vi "CSM Reuse Module.vi"(5 "Init State (\"Macro: Initialize\")":string="Macro: Initialize", 7 "Name (\"\" to Use UUID)":string="Reuse Module") -> ()   [LabVIEW 2017, in "1. Create a reuse Module.lvlib"]
doc: "------------- lvcsm -------------\n[CSMStates]\nItem 0 = \"Event Structure\"\nItem 1 = \"Idle\"\nItem 2 = \"CSM Documentation\"\nItem 3 = \"VI Reference\"\nItem 4 = \"Error Handler\"\nItem 5 = \"Critical Error\"\nItem 6 = \"Target Error\"\nItem 7 = \"Target Timeout Error\"\nItem 8 = \"Async Response\"\nItem 9 = \"Response\"\nItem 10 = \"Async Message Posted\"\nItem 11 = \"Initialize Core Data\"\nItem 12 = \"Exit\"\nItem 13 = \"Data: Initialize\"\nItem 14 = \"Data: Cleanup\"\nItem 15 = \"Events: Register\"\nItem 16 = \"Events: Unregister\"\nItem 17 = \"UI: Initialize\"\nItem 18 = \"UI: Cursor Set\"\nItem 19 = \"UI: Front Panel State\"\nItem 20 = \"Macro: Initialize\"\nItem 21 = \"Macro: Exit\"\nItem 22 = \"API: Start\"\nItem 23 = \"API: Stop\"\nItem 24 = \"API: Set Level\"\nItem 25 = \"API: Get Level\"\nItem 26 = \"DoSth: Check If Greater than 0.5\"\n\n[CSMStatus]\nItem 0 = \"Error Occurred@Error Handler\"\nItem 1 = \"Check Started@API: Start\"\nItem 2 = \"Check Stoppped@API: Stop\""
uses:
  1. Create a reuse Module.lvlib
  user.lib/_NEVSTOP/Communicable State Machine(CSM)/AdvanceAPI/CSM - Break Down Multiple States String.vi
  user.lib/_NEVSTOP/Communicable State Machine(CSM)/AdvanceAPI/CSM - Compact Multiple States.vi
  user.lib/_NEVSTOP/Communicable State Machine(CSM)/AdvanceAPI/CSM - Make String Arguments Safe.vi
  user.lib/_NEVSTOP/Communicable State Machine(CSM)/AdvanceAPI/CSM - Keywords.vi
  user.lib/_NEVSTOP/Communicable State Machine(CSM)/Communicable State Machine.lvlib
panel:
  in  "Level":dbl=0.5 min=0.0 max=1.0 step=0.1 format="%#_13g"
  in  "Stop":bool
  in  "Start":bool
  out "publish status":bool
  out "Random":dbl
  out "State History":string
  # "Creating a reusable module typically does not require message interaction with other modules; it only needs to provide an external interface and publish the state of the module. Therefore, as long as these two aspects are clearly described, one can call the reusable module without understanding its internal implementation details. \n\nIn CSM modules, all cases can be considered as messages for invocation, but it is recommended to use API category as external interfaces. When sending status updates, notify external entities of changes by sending either Status or Interrupt Status. \n\nThe core functionality of this module is to randomly generate data every second and compare it with a threshold value.\n\nAPI: \n1. API: Set Level, with the parameter as a DBL string. Functionality: Configure threshold value.\n2. API: Get Level, without any parameters. Functionality: Retrieve current threshold configuration.\n3. API: Start, without any parameters. Functionality: Initiate random number comparison feature.\n4. API: Stop, without any parameters. Functionality: Cease random number comparison feature.\n\nStatus:\n1. Status Changed, with the parameter as the value of the random number generated when it exceeds 0.5"
  # "If"
  # ">"
  # ", Then"
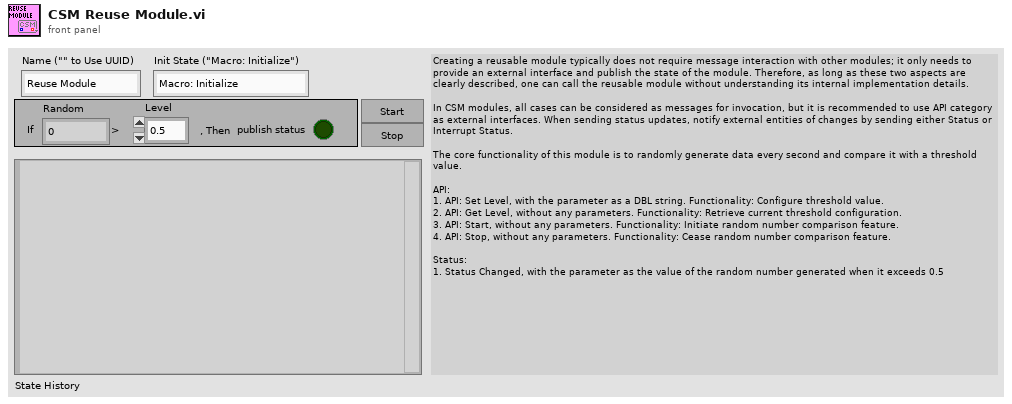
[diagram p1: front panel]
types:
  T1 = enum32{"Invalid", "Standard", "Closed", "Hidden", "Minimized", "Maximized"}
  T2 = enum32{"invalid app kind", "Development System", "Run Time System", "Student Edition", "Embedded LabVIEW", "Evaluation", "Custom"}
  T3 = typedef "Communicable State Machine.lvlib/_CSM_Response Source Message.ctl" = cluster{"‘State":string, "’Arguments":string, "’Error":errorcluster}
  T4 = cluster{"Current VI Reference":refnum<vi>, "Close Panel on Exit?":bool}
  T5 = cluster{"Core":cluster{"Current VI Reference":refnum<vi>, "Close Panel on Exit?":bool}, "Your Boolean data":bool, "Your string data":string, "Level":dbl}
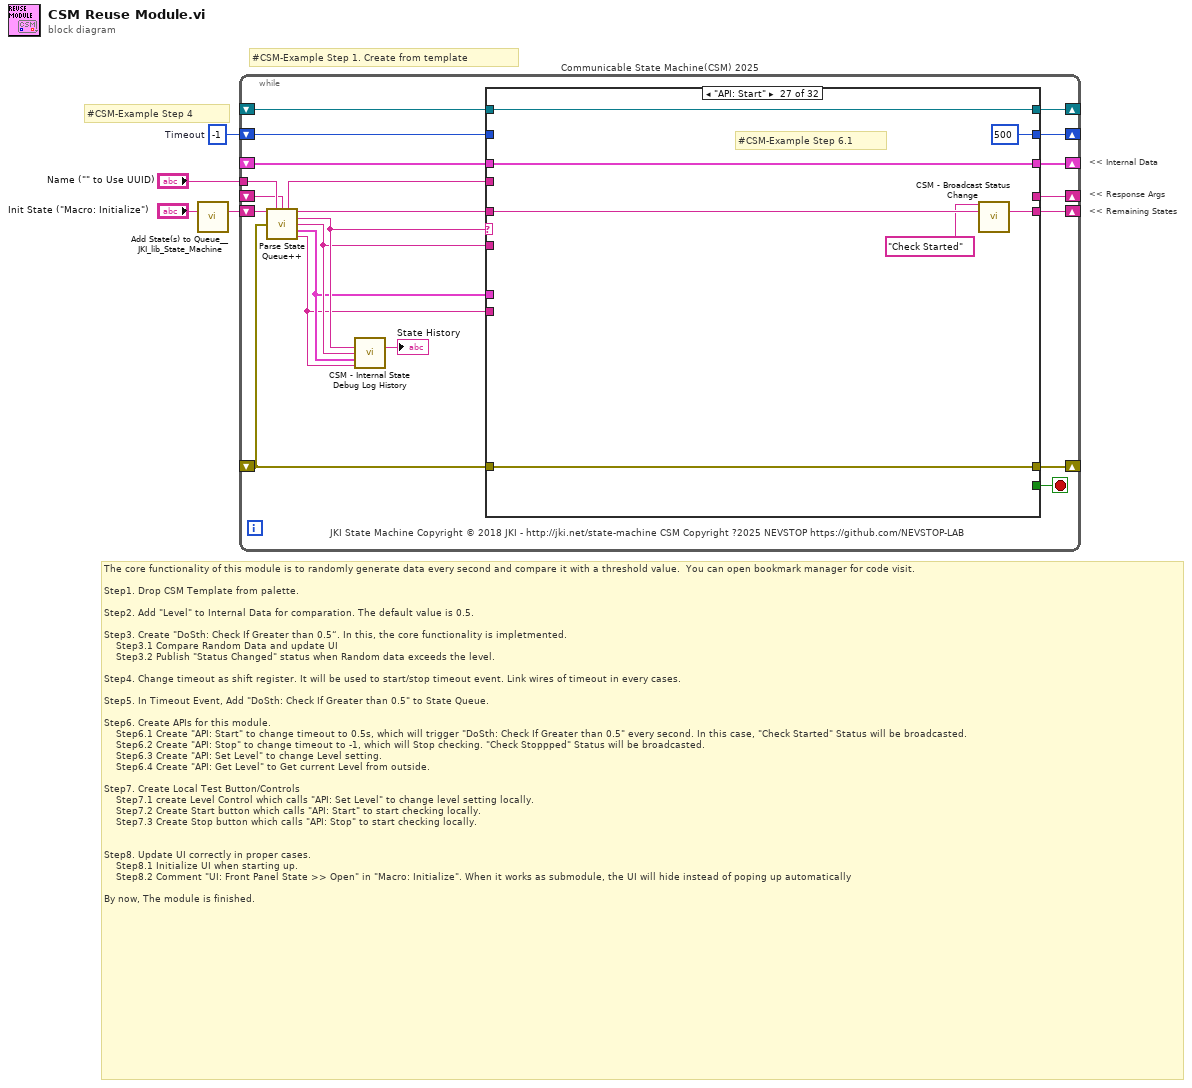
[diagram p0: block diagram]
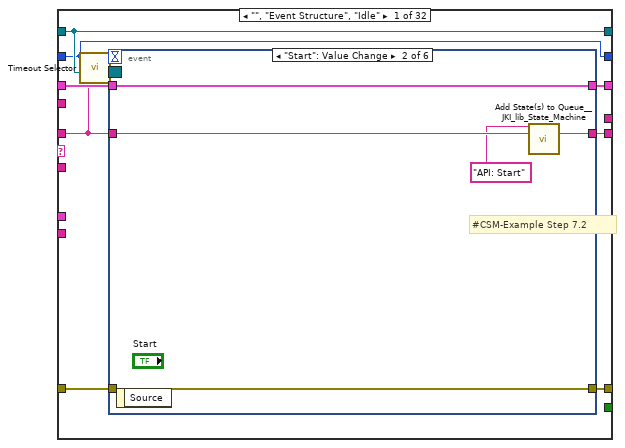
[diagram p2: hidden frame]
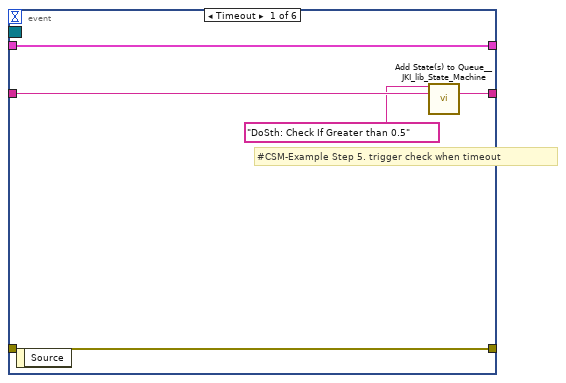
[diagram p3: hidden frame]
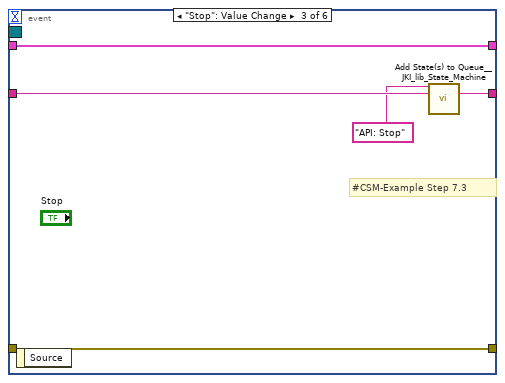
[diagram p4: hidden frame]
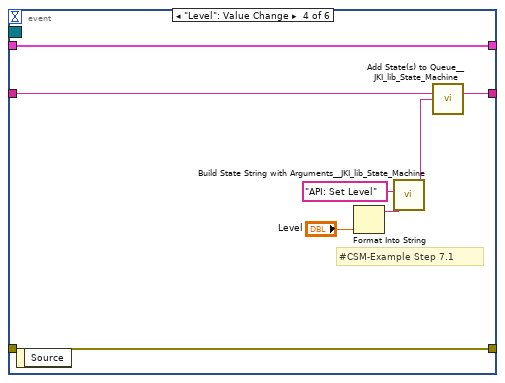
[diagram p5: hidden frame]
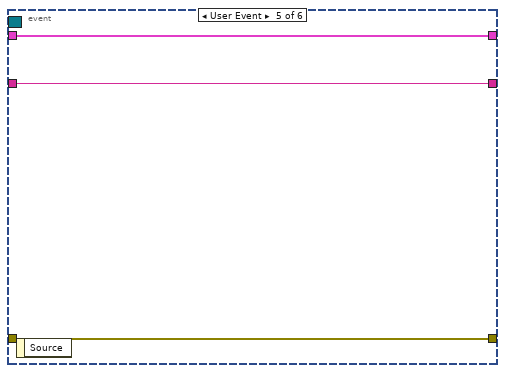
[diagram p6: hidden frame]
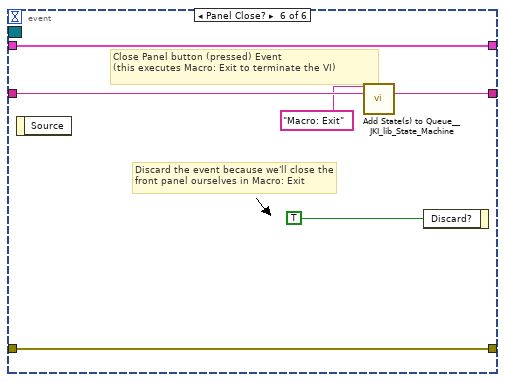
[diagram p7: hidden frame]
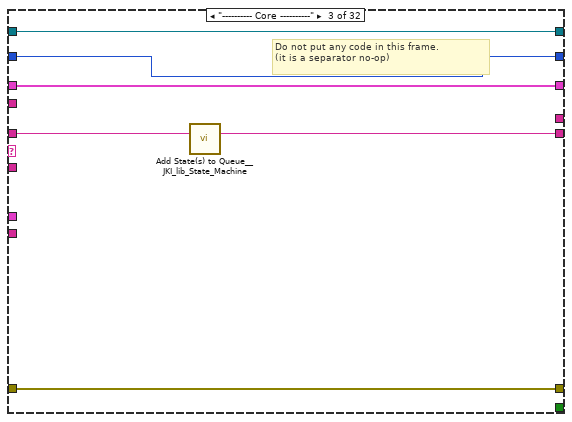
[diagram p9: hidden frame]
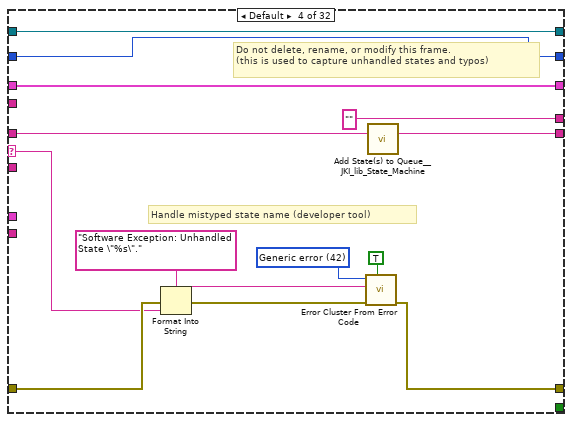
[diagram p10: hidden frame]
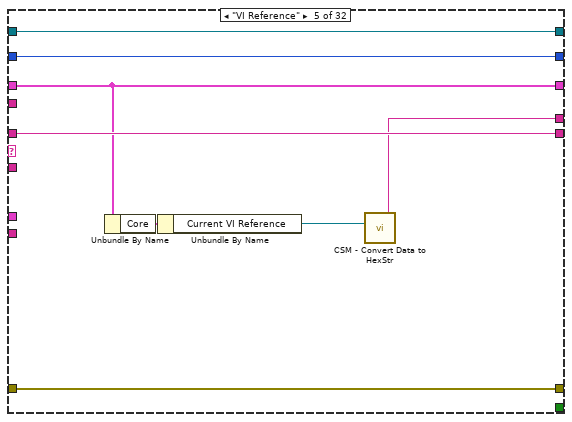
[diagram p11: hidden frame]
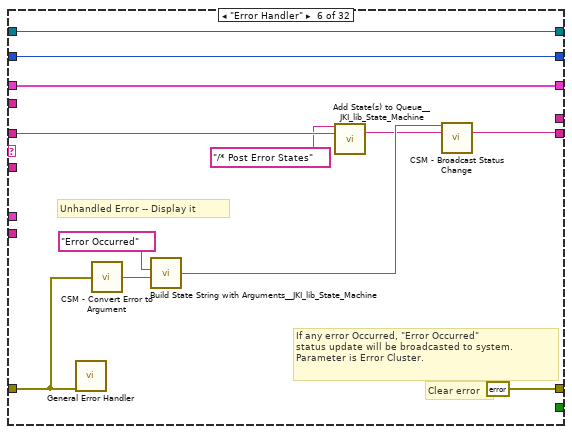
[diagram p12: hidden frame]
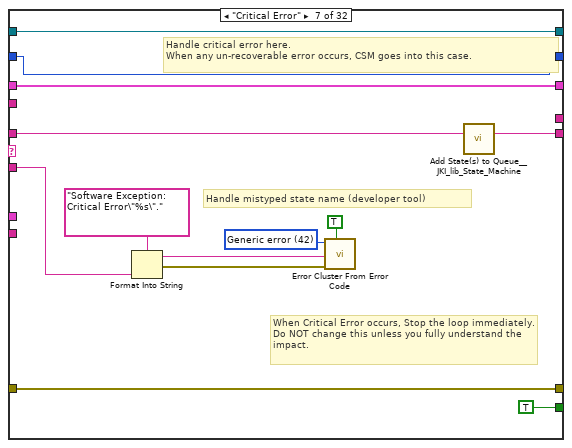
[diagram p13: hidden frame]
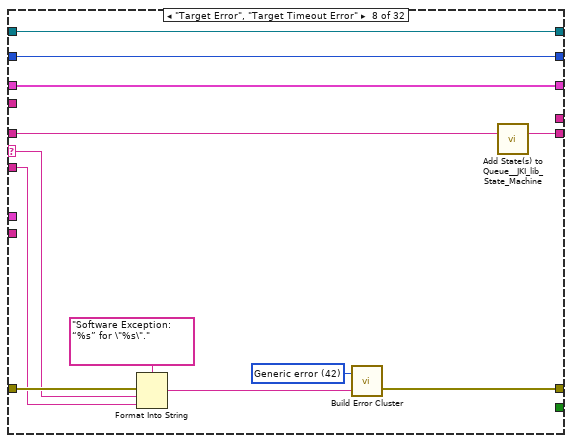
[diagram p14: hidden frame]
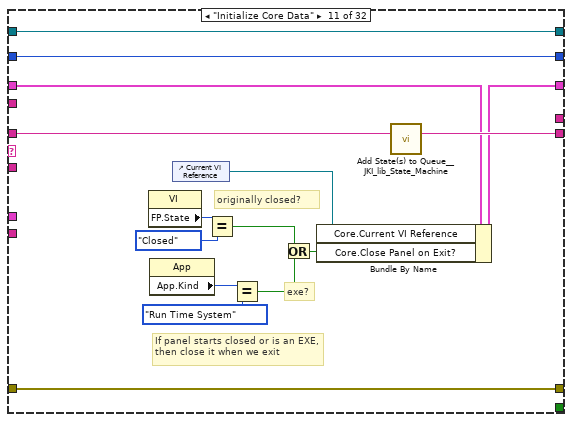
[diagram p17: hidden frame]
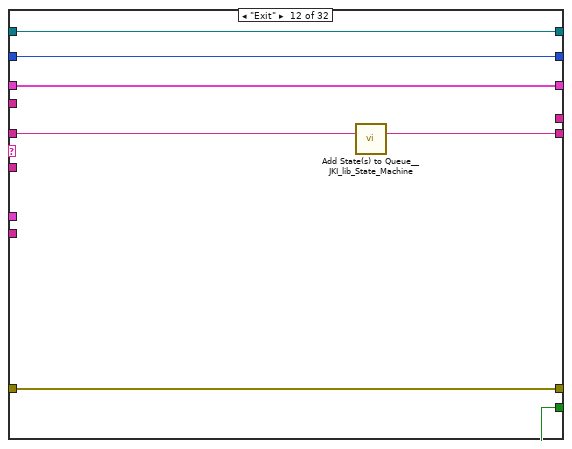
[diagram p18: hidden frame]
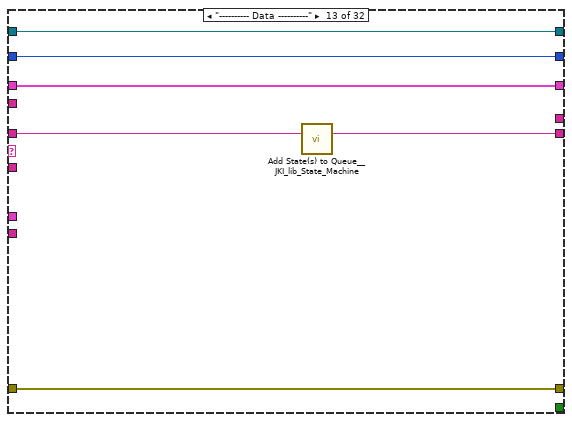
[diagram p19: hidden frame]
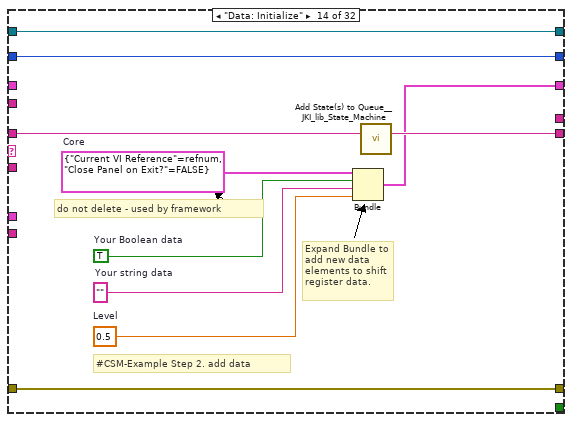
[diagram p20: hidden frame]
diagram:
  w2 = -1  # Timeout
  # "#CSM-Example Step 4"
  # "#CSM-Example Step 1. Create from template"
  # "The core functionality of this module is to randomly generate data every second and compare it with a threshold value.  You can open bookmark manager for code visit.\n\nStep1. Drop CSM Template from palette.\n\nStep2. Add \"Level\" to Internal Data for comparation. The default value is 0.5.\n\nStep3. Create \"DoSth: Check If Greater than 0.5“. In this, the core functionality is impletmented. \n    Step3.1 Compare Random Data and update UI\n    Step3.2 Publish \"Status Changed\" status when Random data exceeds the level.\n\nStep4. Change timeout as shift register. It will be used to start/stop timeout event. Link wires of timeout in every cases. \n\nStep5. In Timeout Event, Add \"DoSth: Check If Greater than 0.5\" to State Queue.\n\nStep6. Create APIs for this module.\n    Step6.1 Create \"API: Start\" to change timeout to 0.5s, which will trigger \"DoSth: Check If Greater than 0.5\" every second. In this case, \"Check Started\" Status will be broadcasted.\n    Step6.2 Create \"API: Stop\" to change timeout to -1, which will Stop checking. \"Check Stoppped\" Status will be broadcasted.\n    Step6.3 Create \"API: Set Level\" to change Level setting.\n    Step6.4 Create \"API: Get Level\" to Get current Level from outside.\n\nStep7. Create Local Test Button/Controls \n    Step7.1 create Level Control which calls \"API: Set Level\" to change level setting locally.\n    Step7.2 Create Start button which calls \"API: Start\" to start checking locally.\n    Step7.3 Create Stop button which calls \"API: Stop\" to start checking locally.\n    \n\nStep8. Update UI correctly in proper cases.\n    Step8.1 Initialize UI when starting up.\n    Step8.2 Comment \"UI: Front Panel State >> Open\" in \"Macro: Initialize\". When it works as submodule, the UI will hide instead of poping up automatically\n\nBy now, The module is finished."
  # "<< Internal Data"
  # "<< Response Args"
  # "<< Remaining States"
  n1 = call <vilib>:"Add State(s) to Queue__JKI_lib_State_Machine.vi"("State(s) in (\"\")"="Init State (\"Macro: Initialize\")") -> ("States Out"=w4:string)  [unwired: 14 in]
  n2 = while "Communicable State Machine(CSM) 2025" {
    shift-right: [w20] -> _
    shift-left: _ -> [w19]
    shift-right: [w23] -> _
    shift-left: _ -> [w18]
    shift-right: [w22] -> _
    shift-left: w4 -> [w24]
    tunnel: "Name (\"\" to Use UUID)" -> [w14]
    shift-right: [w17] -> _
    shift-left: _ -> [w8]
    shift-right: [w16] -> _
    shift-left: _ -> [w15]
    shift-right: [w6] -> _
    shift-left: w2 -> [w7]
    stop <- w21 stop-if-true
    # "JKI State Machine Copyright © 2018 JKI - http://jki.net/state-machine CSM Copyright ?2025 NEVSTOP https://github.com/NEVSTOP-LAB"
    n3 = call "Parse State Queue++.vi"("State Queue"=w24, "Name (\"\" to Use UUID)"=w14, "Response Arguments"=w8, "Previous Error"=w18) -> ("Name Used"=w9:string, "Remaining States"=w25:string, "Current State"=w13:string, "Arguments"=w12:string, ">> Response Source Message >>"=w11:T3, ">> Source CSM >>"=w10:string)  [unwired: 6 in]
    n4 = call "CSM - Internal State Debug Log History.vi"("State"=w13, "Arguments (\"\")"=w12, ">> Response Source Message >>"=w11, "Source (\"\")"=w10) -> ("Debug Log"=→"State History":string)  [unwired: 11 in]
    n5 = case shown="\"API: Start\"" w13 {
      selector: w13 -> [_ _ _ w81 _ _ _ w126 _ _ _ _ _ _ _ _ _ _ _ _ _ _ _ _ _ _ _ _ _ _ _ _]
      tunnel: w25 -> [w27 w70 w77 w85 w98 w111 w122 w128 w140 w145 w161 w168 w174 w184 w192 w198 w205 w210 w217 w224 w232 w249 w320 w327 w339 w343 w350 w357 w365 w372 w379 w393]
      tunnel: w12 -> [_ _ _ _ _ _ w115 w127 _ _ _ _ _ _ _ _ _ _ _ _ w227 w243 _ _ _ _ _ _ w360 _ _ _]
      tunnel: w19 -> [w33 w69 w74 w83 w97 w109 w123 w130 w139 w144 w154 w166 w171 _ w187 w195 w204 w209 w214 w219 w230 w245 w317 w324 w336 w342 w349 w356 w364 w369 w376 w384]
      tunnel: [w32 w71 w75 w87 w99 errorcluster {"status"=FALSE, "code"=0, "source"=""} ("error out") w124 w133 w141 w146 w158 w165 w172 w181 w188 w196 w200 w208 w215 w222 w228 w246 w318 w325 w337 w344 w351 w358 w366 w373 w377 w391] -> w23
      tunnel: w18 -> [w31 w71 w75 w86 w99 w100 w124 w132 w141 w146 w158 w165 w172 w181 w189 w196 _ w211 w215 w222 w229 w247 w318 w325 w337 w344 w351 w358 w366 w373 w377 w391]
      tunnel: [w34 w70 w76 w84 w98 w102 w121 w131 w140 w145 w160 w167 w173 w183 w191 w197 w205 w210 w216 w223 w231 w248 w319 w326 w338 w343 w346 w353 w365 w372 w378 w392] -> w22
      tunnel: [_ _ _ _ _ _ TRUE _ _ _ _ TRUE _ _ _ _ _ _ _ _ _ _ _ _ _ _ _ _ _ _ _ _] -> w21
      tunnel: [w30 w69 w74 w83 w97 w109 w123 w130 w139 w144 w159 w166 w171 w182 w187 w195 w204 w209 w214 w219 w230 w245 w317 w324 w336 w342 w349 w356 w361 w369 w376 w384] -> w20
      tunnel: w7 -> [w26 w67 w72 w78 w95 w101 w112 w125 w137 w142 w147 w162 w169 w176 w185 w193 w199 w206 w212 w220 w225 w241 w315 w321 w328 w340 _ _ w362 w370 w374 w385]
      tunnel: w10 -> [_ _ _ _ _ _ _ _ _ _ _ _ _ _ _ _ _ _ _ _ _ _ _ _ _ _ _ _ _ _ _ _]
      tunnel: w11 -> [_ _ _ _ _ _ _ _ _ _ _ _ _ _ _ _ _ _ _ _ _ _ _ _ _ _ _ _ _ _ _ _]
      tunnel: [_ _ _ "" w92 _ _ _ _ _ _ _ _ _ _ _ _ _ _ _ _ _ _ _ _ _ _ _ _ w367 _ _] -> w17
      tunnel: [w29 w68 w73 w79 w96 w107 w113 w129 w138 w143 w148 w163 w170 w177 w186 w194 w203 w207 w213 w221 w226 w242 w316 w322 w329 w341 w348 w355 w363 w371 w375 w390] -> w16
      tunnel: w15 -> [w29 w68 w73 w79 w96 w107 w113 w129 w138 w143 w148 w163 w170 w177 w186 w194 _ w207 w213 w221 w226 w242 w316 w322 w329 w341 w348 w355 w363 w371 w375 w390]
      tunnel: w9 -> [_ _ _ _ _ _ _ _ _ _ _ _ _ _ _ _ w202 _ _ _ _ _ _ _ _ _ _ _ _ _ _ _]
      tunnel: [w26 w67 w72 w78 w95 w101 w112 w125 w137 w142 w147 w162 w169 w176 w185 w193 w199 w206 w212 w220 w225 w241 w315 w321 w328 w340 500 ("Timeout") -1 ("Timeout") w362 w370 w374 w385] -> w6
      frame "", "Event Structure", "Idle" {
        n6 = call "Timeout Selector.vi"("Remaining States"=w27, "Timeout Expected"=w26) -> ("Timeout"=w28:i32)  [unwired: 5 in]
        n7 = event shown="[1] \"Start\": Value Change" {
          selector: w29 -> [_ _ _ _ _ _]
          dyn-events: _ -> [_ _ _ _ _ _]
          timeout: w28 -> [_ _ _ _ _ _]
          tunnel: w27 -> [w39 w44 w49 w55 w59 w66]
          tunnel: [w38 w43 w48 w54 w59 w65] -> w34
          tunnel: w33 -> [w36 w41 w46 w56 w60 w63]
          tunnel: [w37 w42 w47 w57 w58 w64] -> w32
          tunnel: w31 -> [w37 w42 w47 w57 w58 w64]
          tunnel: [w36 w41 w46 w56 w60 w63] -> w30
          event Timeout {
            # "#CSM-Example Step 5. trigger check when timeout"
            n8 = event-data() -> ()  [unwired: 1 in, 1 out]
            n9 = call <vilib>:"Add State(s) to Queue__JKI_lib_State_Machine.vi"("State(s) in Front (\"\")"="DoSth: Check If Greater than 0.5" ("State(s) in Front (\"\")"), "State(s) in (\"\")"=w39) -> ("States Out"=w38:string)  [unwired: 13 in]
          }
          event "Start": Value Change {
            # "#CSM-Example Step 7.2"
            n10 = event-data() -> ()  [unwired: 1 in, 1 out]
            n11 = call <vilib>:"Add State(s) to Queue__JKI_lib_State_Machine.vi"("State(s) in Front (\"\")"="API: Start" ("State(s) in Front (\"\")"), "State(s) in (\"\")"=w44) -> ("States Out"=w43:string)  [unwired: 13 in]
          }
          event "Stop": Value Change {
            # "#CSM-Example Step 7.3"
            n12 = event-data() -> ()  [unwired: 1 in, 1 out]
            n13 = call <vilib>:"Add State(s) to Queue__JKI_lib_State_Machine.vi"("State(s) in Front (\"\")"="API: Stop" ("State(s) in Front (\"\")"), "State(s) in (\"\")"=w49) -> ("States Out"=w48:string)  [unwired: 13 in]
          }
          event "Level": Value Change {
            # "#CSM-Example Step 7.1"
            n14 = event-data() -> ()  [unwired: 1 in, 1 out]
            n15 = Format Into String("Level") -> (resulting string=w50:string)  [unwired: 3 in, 1 out]
            n16 = call <vilib>:"Build State String with Arguments__JKI_lib_State_Machine.vi"("Arguments (\"\")"=w50, "State"="API: Set Level") -> ("State with Arguments"=w53:string)  [unwired: 4 in]
            n17 = call <vilib>:"Add State(s) to Queue__JKI_lib_State_Machine.vi"("State(s) in (\"\")"=w55, "State(s) at Back (\"\")"=w53) -> ("States Out"=w54:string)  [unwired: 13 in]
          }
          event User Event {
            n18 = event-data() -> ()  [unwired: 1 in, 1 out]
          }
          event Panel Close? {
            # "Discard the event because we'll close the front panel ourselves in Macro: Exit"
            # "Close Panel button (pressed) Event\n(this executes Macro: Exit to terminate the VI)"
            n19 = event-data() -> ()  [unwired: 1 in, 1 out]
            n20 = call <vilib>:"Add State(s) to Queue__JKI_lib_State_Machine.vi"("State(s) in Front (\"\")"="Macro: Exit", "State(s) in (\"\")"=w66) -> ("States Out"=w65:string)  [unwired: 13 in]
            n21 = event-data("Discard?"=TRUE) -> ()  [unwired: 1 in, 1 out]
          }
        }
      }
      frame "CSM Documentation" {
        # "#CSM README FIRST\n\nCSM is a LabVIEW application framework that builds upon JKI State Machine (JKISM). It follows the pattern of JKISM and extends the keywords to describe message communication between CSM modules, including concepts such as Sync-Message, Async-Message, Subscription/Unsubscription of status - essential elements for creating reusable code modules. For more information, please visit the CSM wiki: https://github.com/NEVSTOP-LAB/JKI-State-Machine-Plus-Plus/wiki\n\nFor instructions on JKI State Machine, visit: http://jki.net/state-machine/\nFor information about CSM, visit: https://github.com/NEVSTOP-LAB"
        # "CSM Documentation"
      }
      frame "---------- Core ----------" {
        # "Do not put any code in this frame.\n(it is a separator no-op)"
        n22 = call <vilib>:"Add State(s) to Queue__JKI_lib_State_Machine.vi"("State(s) in (\"\")"=w77) -> ("States Out"=w76:string)  [unwired: 14 in]
      }
      frame Default {
        w90 = 42 items=["No error", "Argument error", "Memory is full", "Out of zone", "End of file", "File already open", "Generic file I/O error", "File not found", "File permission error", "Disk is full", "Duplicate path", "Too many files open", "System feature not enabled", "Resource file not found", "Cannot add resource", "Resource not found", "Image not found", "Image memory error", "Pen does not exist", "Config type invalid", "Config token not found", "Config parse error", "Config memory error", "Bad external code format", "Bad external code offset", "External code not present", "Null window", "Destroy window error", "Null menu", "Print aborted", "Bad print record", "Print driver error", "Windows error during printing", "Memory error during printing", "Print dialog error", "Generic print error", "Invalid device refnum", "Device not found", "Device parameter error", "Device unit error", "Cannot open device", "Device call aborted", "Generic error", "Cancelled by user", "Object ID too low", "Object ID too high", "Object not in heap", "Unknown heap", "Unknown object (invalid DefProc)", "Unknown object (DefProc not in table)", "Message out of range", "Invalid (null) method", "Unknown message", "Manager call not supported", "Bad address", "Network operation in progress", "Network operation timed out", "Connection is busy", "Network attribute not supported", "Network error", "Address in use", "System out of memory", "Connection aborted", "Connection refused", "Not connected", "Already connected", "Connection closed", "Initialization error (interapplication manager)", "Bad occurrence", "Wait on unbound occurrence handler", "Occurrence queue overflow", "Datalog type conflict", "Unused", "Unrecognized type (interapplication manager)", "Memory corrupt", "Failed to make temporary DLL", "Old CIN version", "Drag socket not found", "Failed to load drop-object", "Failed to register OLE object", "Failed to release OLE object", "Format specifier type mismatch", "Unknown format specifier", "Too few format specifiers", "Too many format specifiers", "Scan failed", "Newer CIN version", "Error converting to variant", "Runtime menu error", "Password tampered", "Variant attribute not found", "Incompatible variant data type", "Event data is not available", "Event Store is not present", "Occurrence is not found", "Event Queue is not created", "Event info is not available", "Refnum passed is NULL", "Error retrieving Class GUID", "Error retrieving CoClass GUID", "Error retrieving TypeLib GUID.", "Bad built application magic bytes.", "Specific driver is different from the specific driver associated with the Logical Name.", "There is no session opened to the class driver.", "Max Error", "MAX - Error with config objects", "MAX - Error loading configuration", "MAX - Group not supported"]
        # "Do not delete, rename, or modify this frame.\n(this is used to capture unhandled states and typos)"
        # "Handle mistyped state name (developer tool)"
        n23 = Format Into String(format string="Software Exception: Unhandled State \"%s\"." ("message"), error in=w86, w81) -> (resulting string=w89:string, error out=w88:errorcluster)  [unwired: 1 in]
        n24 = call <vilib>:"Error Cluster From Error Code.vi"("show call chain? (False)"=TRUE, "error in (no error)"=w88, "error message (\"\")"=w89, "error code (0)"=w90) -> ("error out"=w87:errorcluster)  [unwired: 5 in]
        n25 = call <vilib>:"Add State(s) to Queue__JKI_lib_State_Machine.vi"("State(s) in (\"\")"=w85) -> ("States Out"=w84:string)  [unwired: 14 in]
      }
      frame "VI Reference" {
        n26 = Unbundle By Name(w97) -> ("Core"=w94:T4)
        n27 = Unbundle By Name(w94) -> ("Current VI Reference"=w93:refnum<vi>)
        n28 = call "CSM - Convert Data to HexStr.vi"("Variant"=w93) -> ("HEX String (0-9,A-F)"=w92:string)  [unwired: 8 in]
      }
      frame "Error Handler" {
        # "If any error Occurred, \"Error Occurred\" \nstatus update will be broadcasted to system.\nParameter is Error Cluster."
        # "Unhandled Error -- Display it"
        # "Clear error"
        n29 = call <vilib>:"General Error Handler.vi"("error in (no error)"=w100) -> ()  [unwired: 10 in, 5 out]
        n30 = call "CSM - Convert Error to Argument.vi"("Error"=w100) -> ("Argument"=w105:string)  [unwired: 4 in]
        n31 = call <vilib>:"Build State String with Arguments__JKI_lib_State_Machine.vi"("Arguments (\"\")"=w105, "State"="Error Occurred" ("Status with Arguments")) -> ("State with Arguments"=w104:string)  [unwired: 4 in]
        n32 = call <vilib>:"Add State(s) to Queue__JKI_lib_State_Machine.vi"("State(s) in Front (\"\")"="/* Post Error States", "State(s) in (\"\")"=w111) -> ("States Out"=w103:string)  [unwired: 13 in]
        n33 = call "CSM - Broadcast Status Change.vi"("Status With Arguments"=w104, "State Queue"=w103) -> ("Remaining States"=w102:string)  [unwired: 13 in]
      }
      frame "Critical Error" {
        w119 = 42 items=["No error", "Argument error", "Memory is full", "Out of zone", "End of file", "File already open", "Generic file I/O error", "File not found", "File permission error", "Disk is full", "Duplicate path", "Too many files open", "System feature not enabled", "Resource file not found", "Cannot add resource", "Resource not found", "Image not found", "Image memory error", "Pen does not exist", "Config type invalid", "Config token not found", "Config parse error", "Config memory error", "Bad external code format", "Bad external code offset", "External code not present", "Null window", "Destroy window error", "Null menu", "Print aborted", "Bad print record", "Print driver error", "Windows error during printing", "Memory error during printing", "Print dialog error", "Generic print error", "Invalid device refnum", "Device not found", "Device parameter error", "Device unit error", "Cannot open device", "Device call aborted", "Generic error", "Cancelled by user", "Object ID too low", "Object ID too high", "Object not in heap", "Unknown heap", "Unknown object (invalid DefProc)", "Unknown object (DefProc not in table)", "Message out of range", "Invalid (null) method", "Unknown message", "Manager call not supported", "Bad address", "Network operation in progress", "Network operation timed out", "Connection is busy", "Network attribute not supported", "Network error", "Address in use", "System out of memory", "Connection aborted", "Connection refused", "Not connected", "Already connected", "Connection closed", "Initialization error (interapplication manager)", "Bad occurrence", "Wait on unbound occurrence handler", "Occurrence queue overflow", "Datalog type conflict", "Unused", "Unrecognized type (interapplication manager)", "Memory corrupt", "Failed to make temporary DLL", "Old CIN version", "Drag socket not found", "Failed to load drop-object", "Failed to register OLE object", "Failed to release OLE object", "Format specifier type mismatch", "Unknown format specifier", "Too few format specifiers", "Too many format specifiers", "Scan failed", "Newer CIN version", "Error converting to variant", "Runtime menu error", "Password tampered", "Variant attribute not found", "Incompatible variant data type", "Event data is not available", "Event Store is not present", "Occurrence is not found", "Event Queue is not created", "Event info is not available", "Refnum passed is NULL", "Error retrieving Class GUID", "Error retrieving CoClass GUID", "Error retrieving TypeLib GUID.", "Bad built application magic bytes.", "Specific driver is different from the specific driver associated with the Logical Name.", "There is no session opened to the class driver.", "Max Error", "MAX - Error with config objects", "MAX - Error loading configuration", "MAX - Group not supported"]
        # "Handle critical error here.\nWhen any un-recoverable error occurs, CSM goes into this case."
        # "When Critical Error occurs, Stop the loop immediately. Do NOT change this unless you fully understand the impact."
        # "Handle mistyped state name (developer tool)"
        n34 = Format Into String(format string="Software Exception: Critical Error\"%s\"." ("message"), w115) -> (resulting string=w118:string, error out=w117:errorcluster)  [unwired: 2 in]
        n35 = call <vilib>:"Error Cluster From Error Code.vi"("show call chain? (False)"=TRUE, "error in (no error)"=w117, "error message (\"\")"=w118, "error code (0)"=w119) -> ()  [unwired: 5 in, 1 out]
        n36 = call <vilib>:"Add State(s) to Queue__JKI_lib_State_Machine.vi"("State(s) in (\"\")"=w122) -> ("States Out"=w121:string)  [unwired: 14 in]
      }
      frame "Target Error", "Target Timeout Error" {
        w135 = 42 items=["No error", "Argument error", "Memory is full", "Out of zone", "End of file", "File already open", "Generic file I/O error", "File not found", "File permission error", "Disk is full", "Duplicate path", "Too many files open", "System feature not enabled", "Resource file not found", "Cannot add resource", "Resource not found", "Image not found", "Image memory error", "Pen does not exist", "Config type invalid", "Config token not found", "Config parse error", "Config memory error", "Bad external code format", "Bad external code offset", "External code not present", "Null window", "Destroy window error", "Null menu", "Print aborted", "Bad print record", "Print driver error", "Windows error during printing", "Memory error during printing", "Print dialog error", "Generic print error", "Invalid device refnum", "Device not found", "Device parameter error", "Device unit error", "Cannot open device", "Device call aborted", "Generic error", "Cancelled by user", "Object ID too low", "Object ID too high", "Object not in heap", "Unknown heap", "Unknown object (invalid DefProc)", "Unknown object (DefProc not in table)", "Message out of range", "Invalid (null) method", "Unknown message", "Manager call not supported", "Bad address", "Network operation in progress", "Network operation timed out", "Connection is busy", "Network attribute not supported", "Network error", "Address in use", "System out of memory", "Connection aborted", "Connection refused", "Not connected", "Already connected", "Connection closed", "Initialization error (interapplication manager)", "Bad occurrence", "Wait on unbound occurrence handler", "Occurrence queue overflow", "Datalog type conflict", "Unused", "Unrecognized type (interapplication manager)", "Memory corrupt", "Failed to make temporary DLL", "Old CIN version", "Drag socket not found", "Failed to load drop-object", "Failed to register OLE object", "Failed to release OLE object", "Format specifier type mismatch", "Unknown format specifier", "Too few format specifiers", "Too many format specifiers", "Scan failed", "Newer CIN version", "Error converting to variant", "Runtime menu error", "Password tampered", "Variant attribute not found", "Incompatible variant data type", "Event data is not available", "Event Store is not present", "Occurrence is not found", "Event Queue is not created", "Event info is not available", "Refnum passed is NULL", "Error retrieving Class GUID", "Error retrieving CoClass GUID", "Error retrieving TypeLib GUID.", "Bad built application magic bytes.", "Specific driver is different from the specific driver associated with the Logical Name.", "There is no session opened to the class driver.", "Max Error", "MAX - Error with config objects", "MAX - Error loading configuration", "MAX - Group not supported"]
        n37 = Format Into String(format string="Software Exception: “%s” for \"%s\"." ("message"), error in=w132, w126, w127) -> (resulting string=w134:string)  [unwired: 1 in, 1 out]
        n38 = call "Build Error Cluster.vi"("String to Prepend to Source (\"\")"=w134, "Code"=w135) -> ("error out"=w133:errorcluster)
        n39 = call <vilib>:"Add State(s) to Queue__JKI_lib_State_Machine.vi"("State(s) in (\"\")"=w128) -> ("States Out"=w131:string)  [unwired: 14 in]
      }
      frame "Async Response", "Response" {
        # "Handle Async-call Response (\"Async Response\" for ->)"
        # "Handle Sync-call Response (\"Response\" for @)"
        # "After Message is executed, CSM goes to this state for receive the response. \n    For Async Message(->), \"Async Response\" is used. This CSM will goes to \"Async Message Posted\" immediately and receive the \"Async Response\" after the callee finishes the message.\n    For Sync Message(@),  This CSM will wait until the message is done and immediately goes to \"Response\""
      }
      frame "Async Message Posted" {
        # "Handle post action for async message (->)."
        # "After Async Message is posted (->), CSM goes to this state for post-action. You can use Argument - State to tell which Async Message is called."
      }
      frame "Initialize Core Data" {
        # "originally closed?"
        # "exe?"
        # "If panel starts closed or is an EXE, then close it when we exit"
        n40 = property class="VI"() -> ("FP.State"=w151:T1)  [unwired: 2 in, 2 out]
        n41 = property class="App"() -> ("App.Kind"=w157:T2)  [unwired: 2 in, 2 out]
        n42 = control-ref of="Current VI Reference"() -> (w152:refnum<vi>)
        n43 = Equal?(x=w151, y=T1."Closed" ("Front Panel Window:State")) -> (x = y?=w149:bool)
        n44 = Equal?(x=w157, y=T2."Run Time System" ("Application:Kind")) -> (x = y?=w155:bool)
        n45 = Or(x=w149, y=w155) -> (x .or. y?=w153:bool)
        n46 = Bundle By Name(cluster=w154, "Core.Current VI Reference"=w152, "Core.Close Panel on Exit?"=w153) -> (w159:T5)
        n47 = call <vilib>:"Add State(s) to Queue__JKI_lib_State_Machine.vi"("State(s) in (\"\")"=w161) -> ("States Out"=w160:string)  [unwired: 14 in]
      }
      frame "Exit" {
        n48 = call <vilib>:"Add State(s) to Queue__JKI_lib_State_Machine.vi"("State(s) in (\"\")"=w168) -> ("States Out"=w167:string)  [unwired: 14 in]
      }
      frame "---------- Data ----------" {
        n49 = call <vilib>:"Add State(s) to Queue__JKI_lib_State_Machine.vi"("State(s) in (\"\")"=w174) -> ("States Out"=w173:string)  [unwired: 14 in]
      }
      frame "Data: Initialize" {
        w175 = 0.5  # Level
        w178 = T4 {"Current VI Reference"=refnum, "Close Panel on Exit?"=FALSE}  # Core
        w180 = TRUE  # Your Boolean data
        w179 = ""  # Your string data
        # "#CSM-Example Step 2. add data"
        # "do not delete - used by framework"
        # "Expand Bundle to add new data elements to shift register data."
        n50 = Bundle("Core"=w178, "Your Boolean data"=w180, "Your string data"=w179, "Level"=w175) -> (w182:T5)  [unwired: 1 in]
        n51 = call <vilib>:"Add State(s) to Queue__JKI_lib_State_Machine.vi"("State(s) in (\"\")"=w184) -> ("States Out"=w183:string)  [unwired: 14 in]
      }
      frame "Data: Cleanup" {
        n52 = Unbundle By Name(w187) -> ("Core.Current VI Reference"=w190:refnum<vi>)
        n53 = Close Reference(reference=w190, error in (no error)=w189) -> (error out=w188:errorcluster)
        n54 = call <vilib>:"Add State(s) to Queue__JKI_lib_State_Machine.vi"("State(s) in (\"\")"=w192) -> ("States Out"=w191:string)  [unwired: 14 in]
      }
      frame "---------- Events ----------" {
        n55 = call <vilib>:"Add State(s) to Queue__JKI_lib_State_Machine.vi"("State(s) in (\"\")"=w198) -> ("States Out"=w197:string)  [unwired: 14 in]
      }
      frame "Events: Register" {
        # "Register message event to break Waiting in Event structure."
        n56 = call "CSM - Get New State Notifier Event.vi"("Name (\"\" to Use UUID) In"=w202) -> ("error out"=w200:errorcluster, "New State Notifier Event"=w201:refnum<user-event>)  [unwired: 9 in]
        n57 = register-events(w201) -> (reference out=w203:refnum<event-registration>)  [unwired: 2 in, 1 out]
      }
      frame "Events: Unregister" {
        n58 = Unregister For Events(event registration refnum=w207, error in=w211) -> (error out=w208:errorcluster)
      }
      frame "---------- UI ----------" {
        n59 = call <vilib>:"Add State(s) to Queue__JKI_lib_State_Machine.vi"("State(s) in (\"\")"=w217) -> ("States Out"=w216:string)  [unwired: 14 in]
      }
      frame "UI: Initialize" {
        # "#CSM-Example Step 8.1"
        n60 = Unbundle By Name(w219) -> ("Level"=w218:dbl)
        n61 = local write "Level"(w218) -> ()
        n62 = call <vilib>:"Add State(s) to Queue__JKI_lib_State_Machine.vi"("State(s) in (\"\")"=w224) -> ("States Out"=w223:string)  [unwired: 14 in]
      }
      frame "UI: Cursor Set" {
        # "Argument"
        n63 = disable-structure shown="TARGET_TYPE!=Windows" {
          disable-tunnel: w229 -> [w235 w240]
          disable-tunnel: [w234 w240] -> w228
          disable-tunnel: w227 -> [w233 _]
          frame condition #0 (active) {
            n64 = case shown="\"Idle\", Default" w233 {
              tunnel: w235 -> [w237 w239]
              tunnel: [w236 w238] -> w234
              frame "Idle", Default {
                n65 = call <vilib>:"Unset Busy.vi"("error in (no error)"=w237) -> ("error out"=w236:errorcluster)  [unwired: 10 in]
              }
              frame "Busy" {
                n66 = call <vilib>:"Set Busy.vi"("error in (no error)"=w239) -> ("error out"=w238:errorcluster)  [unwired: 9 in, 1 out]
              }
            }
          }
          frame condition #1 {
          }
        }
        n67 = call <vilib>:"Add State(s) to Queue__JKI_lib_State_Machine.vi"("State(s) in (\"\")"=w232) -> ("States Out"=w231:string)  [unwired: 14 in]
      }
      frame "UI: Front Panel State" {
        # "Argument"
        n68 = Unbundle By Name(w245) -> ("Core.Current VI Reference"=w244:refnum<vi>)
        n69 = call <vilib>:"Add State(s) to Queue__JKI_lib_State_Machine.vi"("State(s) in (\"\")"=w249) -> ("States Out"=w248:string)  [unwired: 14 in]
        n70 = case shown="\"Close\", \"Closed\"" w243 {
          tunnel: w247 -> [w255 w270 w281 w294 w307]
          tunnel: [w257 w271 w283 w296 w309] -> w246
          tunnel: w244 -> [w256 w268 w282 w295 w308]
          frame "Open", "Standard", Default {
            w250 = T1."Standard" ("State")
            n71 = property class="VI"(reference=w256, error in=w255) -> (reference out=w253:refnum<vi>, error out=w254:errorcluster, "FP.State"=w252:T1)
            n72 = Not Equal?(x=w252, y=w250) -> (x != y?=w251:bool)
            n73 = case shown="True" w251 {
              tunnel: [w261 w263] -> w257
              tunnel: w254 -> [w260 w263]
              tunnel: w253 -> [w259 _]
              tunnel: w250 -> [w258 _]
              frame True {
                n74 = invoke class="VI" method="FP.Open"(reference=w259, error in=w260, "Activate"=TRUE, "State"=w258) -> (error out=w261:errorcluster)  [unwired: 1 in, 4 out]
              }
              frame False {
              }
            }
          }
          frame "Close", "Closed" {
            n75 = property class="VI"(reference=w268, error in=w270) -> (reference out=w267:refnum<vi>, error out=w269:errorcluster, "FP.State"=w265:T1)
            n76 = Not Equal?(x=w265, y=T1."Closed" ("Front Panel Window:State")) -> (x != y?=w264:bool)
            n77 = case shown="True" w264 {
              tunnel: [w272 w275] -> w271
              tunnel: w269 -> [w272 w274]
              tunnel: w267 -> [_ w273]
              frame False {
              }
              frame True {
                n78 = invoke class="VI" method="FP.Close"(reference=w273, error in=w274) -> (error out=w275:errorcluster)  [unwired: 1 in, 2 out]
              }
            }
          }
          frame "Hidden", "Hide" {
            w276 = T1."Hidden" ("State")
            n79 = property class="VI"(reference=w282, error in=w281) -> (reference out=w279:refnum<vi>, error out=w280:errorcluster, "FP.State"=w278:T1)
            n80 = Not Equal?(x=w278, y=w276) -> (x != y?=w277:bool)
            n81 = case shown="True" w277 {
              tunnel: [w287 w288] -> w283
              tunnel: w280 -> [w286 w288]
              tunnel: w279 -> [w285 _]
              tunnel: w276 -> [w284 _]
              frame True {
                n82 = invoke class="VI" method="FP.Open"(reference=w285, error in=w286, "State"=w284) -> (error out=w287:errorcluster)  [unwired: 2 in, 4 out]
              }
              frame False {
              }
            }
          }
          frame "Minimize", "Minimized" {
            w289 = T1."Minimized" ("State")
            n83 = property class="VI"(reference=w295, error in=w294) -> (reference out=w292:refnum<vi>, error out=w293:errorcluster, "FP.State"=w291:T1)
            n84 = Not Equal?(x=w291, y=w289) -> (x != y?=w290:bool)
            n85 = case shown="True" w290 {
              tunnel: [w300 w301] -> w296
              tunnel: w293 -> [w299 w301]
              tunnel: w292 -> [w298 _]
              tunnel: w289 -> [w297 _]
              frame True {
                n86 = invoke class="VI" method="FP.Open"(reference=w298, error in=w299, "State"=w297) -> (error out=w300:errorcluster)  [unwired: 2 in, 4 out]
              }
              frame False {
              }
            }
          }
          frame "Maximize", "Maximized" {
            w302 = T1."Maximized" ("State")
            n87 = property class="VI"(reference=w308, error in=w307) -> (reference out=w305:refnum<vi>, error out=w306:errorcluster, "FP.State"=w304:T1)
            n88 = Not Equal?(x=w304, y=w302) -> (x != y?=w303:bool)
            n89 = case shown="True" w303 {
              tunnel: [w313 w314] -> w309
              tunnel: w306 -> [w312 w314]
              tunnel: w305 -> [w311 _]
              tunnel: w302 -> [w310 _]
              frame True {
                n90 = invoke class="VI" method="FP.Open"(reference=w311, error in=w312, "State"=w310) -> (error out=w313:errorcluster)  [unwired: 2 in, 4 out]
              }
              frame False {
              }
            }
          }
        }
      }
      frame "---------- Macro ----------" {
        n91 = call <vilib>:"Add State(s) to Queue__JKI_lib_State_Machine.vi"("State(s) in (\"\")"=w320) -> ("States Out"=w319:string)  [unwired: 14 in]
      }
      frame "Macro: Initialize" {
        w323 = "Data: Initialize\nInitialize Core Data\nEvents: Register\nUI: Initialize\n//Disable Open front panel to make it running behind\n//UI: Front Panel State >> Open"  # Data: Initialize Initialize Core Data Events: Register UI: Initialize //Disable Open front panel to make it running behind //UI: Front Panel State >> Open
        # "#CSM-Example Step 8.2 Disable Open front panel to make it running behind"
        n92 = call <vilib>:"Add State(s) to Queue__JKI_lib_State_Machine.vi"("State(s) in Front (\"\")"=w323, "State(s) in (\"\")"=w327) -> ("States Out"=w326:string)  [unwired: 13 in]
      }
      frame "Macro: Exit" {
        n93 = Unbundle By Name(w336) -> ("Core.Close Panel on Exit?"=w335:bool)
        n94 = Select(t="UI: Front Panel State >> Close", s=w335, f="") -> (s? t:f=w332:string)
        n95 = call <vilib>:"Add State(s) to Queue__JKI_lib_State_Machine.vi"("State(s) in (\"\")"=w332, "State(s) at Back (\"\")"="Data: Cleanup\nEvents: Unregister\nExit") -> ("States Out"=w330:string)  [unwired: 13 in]
        n96 = call <vilib>:"Add State(s) to Queue__JKI_lib_State_Machine.vi"("State(s) in Front (\"\")"=w330, "State(s) in (\"\")"=w339) -> ("States Out"=w338:string)  [unwired: 13 in]
      }
      frame "---------- API ----------" {
      }
      frame "API: Start" {
        # "#CSM-Example Step 6.1"
        n97 = call "CSM - Broadcast Status Change.vi"("Status With Arguments"="Check Started" ("Status with Arguments"), "State Queue"=w350) -> ("Remaining States"=w346:string)  [unwired: 13 in]
      }
      frame "API: Stop" {
        # "#CSM-Example Step 6.2"
        n98 = call "CSM - Broadcast Status Change.vi"("Status With Arguments"="Check Stoppped" ("Status with Arguments"), "State Queue"=w357) -> ("Remaining States"=w353:string)  [unwired: 13 in]
      }
      frame "API: Set Level" {
        # "#CSM-Example Step 6.3"
        n99 = Fract/Exp String To Number(string=w360) -> (number=w359:dbl)  [unwired: 3 in, 1 out]
        n100 = local write "Level"(w359) -> ()
        n101 = Bundle By Name(cluster=w364, "Level"=w359) -> (w361:T5)
      }
      frame "API: Get Level" {
        # "#CSM-Example Step 6.4"
        n102 = Unbundle By Name(w369) -> ("Level"=w368:dbl)
        n103 = Format Into String(w368) -> (resulting string=w367:string)  [unwired: 3 in, 1 out]
      }
      frame "---------- DoSth ----------" {
        n104 = call <vilib>:"Add State(s) to Queue__JKI_lib_State_Machine.vi"("State(s) in (\"\")"=w379) -> ("States Out"=w378:string)  [unwired: 14 in]
      }
      frame "DoSth: Check If Greater than 0.5" {
        # "#CSM-Example Step 3.2"
        # "#CSM-Example Step 3.1"
        # "#CSM-Example Step 3. Core functionality"
        n105 = Unbundle By Name(w384) -> ("Level"=w383:dbl)
        n106 = Random Number (0-1)() -> (number: 0 to 1=w389:dbl)
        "Random" <- w389
        n107 = Greater?(x=w389, y=w383) -> (0:w386:bool)
        "publish status" <- w386
        n108 = Format Into String(w389) -> (resulting string=w387:string)  [unwired: 3 in, 1 out]
        n109 = call <vilib>:"Build State String with Arguments__JKI_lib_State_Machine.vi"("Arguments (\"\")"=w387, "State"="Status Changed") -> ("State with Arguments"=w381:string)  [unwired: 4 in]
        n110 = call <vilib>:"Add State(s) to Queue__JKI_lib_State_Machine.vi"("State(s) in (\"\")"="Another Status" ("State"), "State(s) at Back (\"\")"=w381) -> ("States Out"=w380:string)  [unwired: 13 in]
        n111 = call "CSM - Broadcast Status Change.vi"("Status With Arguments"=w380, "State Queue"=w393, "Broadcast? (T)"=w386) -> ("Remaining States"=w392:string)  [unwired: 12 in]
      }
    }
  }
